vi "2D array search.vi"(4 "Alternative":string, 6 "Option for alternative":string, 9 "Search For":string, 11 "Input Array":string[][](array[string])) -> (0 "Column":i32, 1 "Row":i32, 3 "element":string)   [LabVIEW 2018]
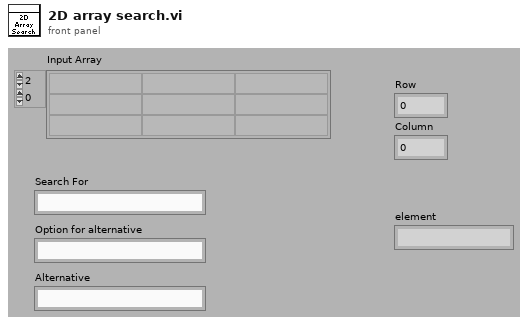
[diagram p1: front panel]
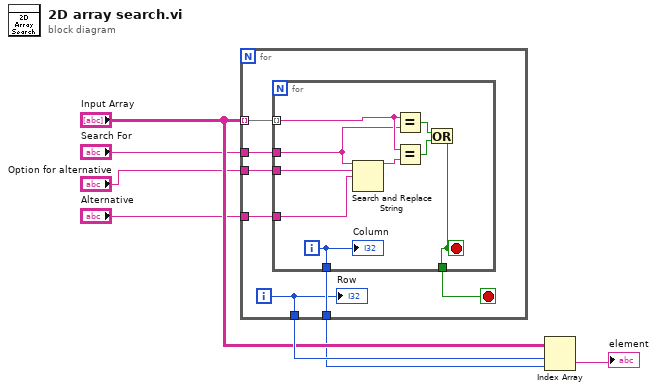
[diagram p0: block diagram]
diagram:
  n1 = for {
    tunnel: "Input Array" -> [w14] mode=indexing
    tunnel: [w11] -> w7
    tunnel: [w13] -> w5
    tunnel: "Search For" -> [w10]
    tunnel: "Option for alternative" -> [w9]
    tunnel: "Alternative" -> [w8]
    i -> [w11]
    stop <- w12 stop-if-true
    n2 = for {
      tunnel: w14 -> [w22] mode=indexing
      tunnel: [w23] -> w13
      tunnel: [w20] -> w12
      tunnel: w10 -> [w17]
      tunnel: w9 -> [w16]
      tunnel: w8 -> [w15]
      i -> [w23]
      stop <- w20 stop-if-true
      n3 = Search and Replace String(input string=w17, search string=w16, replace string=w15) -> (result string=w21:string)  [unwired: 5 in, 3 out]
      n4 = Equal?(x=w22, y=w17) -> (x = y?=w19:bool)
      n5 = Equal?(x=w22, y=w21) -> (x = y?=w18:bool)
      n6 = Or(x=w19, y=w18) -> (x .or. y?=w20:bool)
      "Column" <- w23
    }
    "Row" <- w11
  }
  n7 = Index Array(array="Input Array", index (row)=w7, index (col)=w5) -> (element=→"element":string)
